vi "send.vi"(0 "HGF_SVEvent":refnum<class "HGF_SVEvent.lvclass">, 2 "Object":refnum<class>, 3 "timeout in ms (-1)":i32, 5 "error in (no error)":errorcluster, 9 "mode (Queue)":bool) -> (14 "dup HGF_SVEvent":refnum<class "HGF_SVEvent.lvclass">, 17 "timed out?":bool, 19 "error out":errorcluster)   [LabVIEW 2012, in "HGF_SV.lvlib" / "HGF_SVEvent.lvclass"]
doc: "Send an object.\n\nHint: This is a dynamic dispatch VI to be implemented by the child class."
uses:
  HGF_SVEvent.lvclass
  HGF_BaseClasses/HGF_NetworkVisitor/HGF_NetworkVisitor.lvclass
  HGF_SVEvent.lvclass/HGF_SVEvent.ctl
  HGF_Auxiliary/Severity.ctl
  HGF_Auxiliary/ErrorCode.ctl
  HGF_Auxiliary/HGF_Auxiliary.lvlib
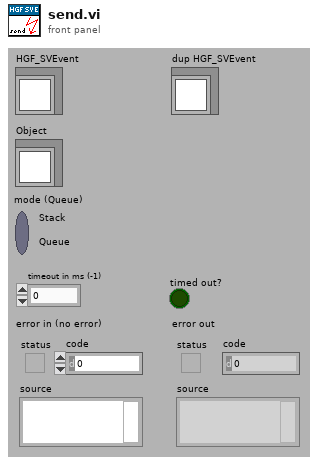
[diagram p1: front panel]
types:
  T1 = typedef "HGF_Auxiliary.lvlib/ErrorCode.ctl" = enum32{"No error", "Function not supported.", "This VI is for friends only.", "Reference object aready exisits.", "Parameter out of range.", "Not a rendezvous.", "Invalid notifier reference.", "Invalid queue reference.", "Self-Test not supported.", "Reset not supported.", "IDN query not supported.", "Error query not supported.", "Incorrect addressee.", "Object already exists.", "No class name specified", "Driver not supported", "Attribute is not writable"}
  T2 = typedef "HGF_Auxiliary.lvlib/Severity.ctl" = enum16{"Info", "Warning", "Fault", "Error", "Fatal"}
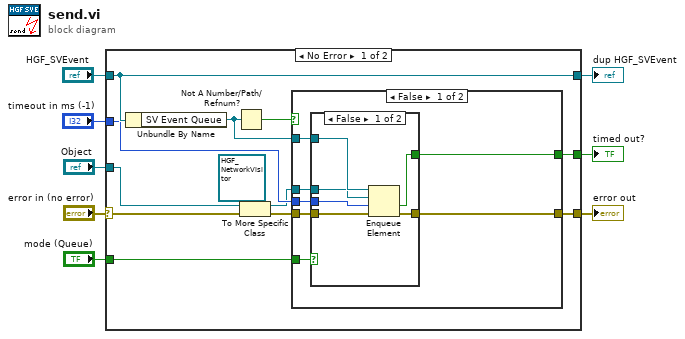
[diagram p0: block diagram]
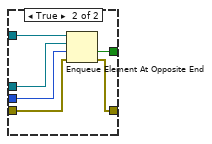
[diagram p2: hidden frame]
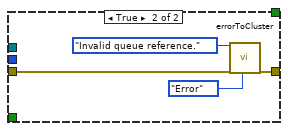
[diagram p3: hidden frame]
diagram:
  n1 = case shown="No Error" "error in (no error)" {
    selector: "error in (no error)" -> [w11 w45]
    tunnel: [w20 w45] -> w5
    tunnel: [w19 _] -> w6
    tunnel: "HGF_SVEvent" -> [w17 w44]
    tunnel: [w17 w44] -> w7
    tunnel: "timeout in ms (-1)" -> [w15 _]
    tunnel: "mode (Queue)" -> [w14 _]
    tunnel: "Object" -> [w12 _]
    frame No Error {
      n2 = Unbundle By Name(w17) -> ("SV Event Queue"=w16:refnum<queue>)
      n3 = Not A Number/Path/Refnum?(number/path/refnum=w16) -> (NaN/Path/Refnum?=w18:bool)
      n4 = To More Specific Class(target class=refnum<class "HGF_NetworkVisitor.lvclass"> refnum ("element"), reference=w12, error in=w11) -> (specific class reference=w9:refnum<class "HGF_NetworkVisitor.lvclass">, error out=w10:errorcluster)
      n5 = case shown="False" w18 {
        tunnel: [w27 w42] -> w20
        tunnel: [w26 _] -> w19
        tunnel: w10 -> [w25 w43]
        tunnel: w16 -> [w24 _]
        tunnel: w15 -> [w23 _]
        tunnel: w14 -> [w22 _]
        tunnel: w9 -> [w21 _]
        frame False {
          n6 = case shown="False" w22 {
            tunnel: [w33 w38] -> w27
            tunnel: [w32 w39] -> w26
            tunnel: w25 -> [w31 w37]
            tunnel: w24 -> [w30 w34]
            tunnel: w23 -> [w29 w36]
            tunnel: w21 -> [w28 w35]
            frame False {
              n7 = Enqueue Element(queue=w30, element=w28, timeout in ms (-1)=w29, error in (no error)=w31) -> (timed out?=w32:bool, error out=w33:errorcluster)  [unwired: 1 out]
            }
            frame True {
              n8 = Enqueue Element At Opposite End(queue=w34, element=w35, timeout in ms (-1)=w36, error in (no error)=w37) -> (timed out?=w39:bool, error out=w38:errorcluster)  [unwired: 1 out]
            }
          }
        }
        frame True {
          n9 = call "errorToCluster.vi"("error code"=ErrorCode."Invalid queue reference." ("HGF_Error"), "error in (no error)"=w43, "severity (Error)"=Severity."Error") -> ("error out"=w42:errorcluster)  [unwired: 2 in, 14 out]
        }
      }
    }
    frame Error {
    }
  }
  "error out" <- w5
  "dup HGF_SVEvent" <- w7
  "timed out?" <- w6
